vi "3kButtonsSys22x22.vi"() -> ()   [LabVIEW 2011]
doc: "3000 buttons from haobo.li@pansino.com.cn\nhttp://www.linkedin.com/pub/haobo-li/17/8a/220\nthanks to\nhttp://www.fatcow.com/free-icons"
panel:
  in  "Pansino 2":bool
  in  "Pansino":bool
  in  "zootool":bool
  in  "zoom_selection":bool
  in  "zoom_refresh":bool
  in  "zoom_out":bool
  in  "zoom_layer":bool
  in  "zoom_last":bool
  in  "zoom_in":bool
  in  "zoom_fit":bool
  in  "zoom_extend":bool
  in  "zoom_actual_equal":bool
  in  "zoom_actual":bool
  in  "zoom":bool
  in  "youtube":bool
  in  "yelp":bool
  in  "yellow_submarine":bool
  in  "yahoo_messenger":bool
  in  "yacht":bool
  in  "xing":bool
  in  "xhtml_valid":bool
  in  "xhtml_go":bool
  in  "xhtml_delete":bool
  in  "xhtml_add":bool
  in  "xhtml":bool
  in  "x_ray":bool
  in  "www_page":bool
  in  "wrench_orange":bool
  in  "wrench":bool
  in  "wrapping_tight":bool
  in  "wrapping_square":bool
  in  "wrapping_magazine":bool
  in  "wrapping_inline":bool
  in  "wrapping_in_front":bool
  in  "wrapping_edit":bool
  in  "wrapping_between":bool
  in  "wrapping_behind":bool
  in  "world_link":bool
  in  "world_go":bool
  in  "world_edit":bool
  in  "world_delete":bool
  in  "world_add":bool
  in  "world":bool
  in  "workspace":bool
  in  "wordpress_blog":bool
  in  "wordpress":bool
  in  "wizard_women":bool
  in  "wizard":bool
  in  "wishlist_add":bool
  in  "winrar_view":bool
  in  "winrar_extract":bool
  in  "winrar_add":bool
  in  "wine_pairings":bool
  in  "windy":bool
  in  "widgets":bool
  in  "widescreen":bool
  in  "whistle":bool
  in  "weight":bool
  in  "weighing_mashine":bool
  in  "webcam_error":bool
  in  "webcam_delete":bool
  in  "webcam_add":bool
  in  "webcam":bool
  in  "web_concierge":bool
  in  "weather_sun":bool
  in  "weather_snow":bool
  in  "weather_rain":bool
  in  "weather_lightning":bool
  in  "weather_cloudy":bool
  in  "weather_clouds":bool
  in  "wand":bool
  in  "wallet":bool
  in  "walk":bool
  in  "vslider":bool
  in  "vrule":bool
  in  "vlc":bool
  in  "visa_electron":bool
  in  "visa_2":bool
  in  "visa":bool
  in  "virus_protection":bool
  in  "virb":bool
  in  "vimeo":bool
  in  "viewstack":bool
  in  "videodisplay":bool
  in  "video_mode":bool
  in  "video":bool
  in  "viddler":bool
  in  "vhs":bool
  in  "vector_delete":bool
  in  "vector_add":bool
  in  "vector":bool
  in  "vdividedbox":bool
  in  "vcard_edit":bool
  in  "vcard_delete":bool
  in  "vcard_add":bool
  in  "vcard":bool
  in  "vbox":bool
  in  "user_zorro":bool
  in  "user_yoda":bool
  in  "user_wicket":bool
  in  "user_waiter_female_black":bool
  in  "user_waiter_female":bool
  in  "user_waiter":bool
  in  "user_viking_female":bool
  in  "user_viking":bool
  in  "user_vietnamese_female":bool
  in  "user_vietnamese":bool
  in  "user_trooper_captain":bool
  in  "user_trooper":bool
  in  "user_swimmer_female":bool
  in  "user_swimmer_black":bool
  in  "user_swimmer":bool
  in  "user_superman":bool
  in  "user_suit":bool
  in  "user_student_female_black":bool
  in  "user_student_female":bool
  in  "user_student_black":bool
  in  "user_student":bool
  in  "user_striper_black":bool
  in  "user_striper":bool
  in  "user_stewardess_black":bool
  in  "user_stewardess":bool
  in  "user_squidward":bool
  in  "user_sponge_bob":bool
  in  "user_spiderman":bool
  in  "user_soldier":bool
  in  "user_silhouette":bool
  in  "user_scream":bool
  in  "user_samurai":bool
  in  "user_sailor_black":bool
  in  "user_sailor":bool
  in  "user_robocop":bool
  in  "user_redskin":bool
  in  "user_red":bool
  in  "user_rambo":bool
  in  "user_racer":bool
  in  "user_r2d2":bool
  in  "user_queen_black":bool
  in  "user_queen":bool
  in  "user_pumpkin":bool
  in  "user_priest_black":bool
  in  "user_priest":bool
  in  "user_policeman_black":bool
  in  "user_policeman":bool
  in  "user_police_female_black":bool
  in  "user_police_female":bool
  in  "user_police_england":bool
  in  "user_plankton":bool
  in  "user_pirate":bool
  in  "user_pilot_civil":bool
  in  "user_pilot":bool
  in  "user_patrick":bool
  in  "user_orange":bool
  in  "user_oldwoman_black":bool
  in  "user_oldwoman":bool
  in  "user_oldman_black":bool
  in  "user_oldman":bool
  in  "user_officer_black":bool
  in  "user_officer":bool
  in  "user_nun_black":bool
  in  "user_nun":bool
  in  "user_nude_female_black":bool
  in  "user_nude_female":bool
  in  "user_nude_black":bool
  in  "user_nude":bool
  in  "user_ninja":bool
  in  "user_muslim_female":bool
  in  "user_muslim":bool
  in  "user_mexican":bool
  in  "user_medical_female_black":bool
  in  "user_medical_female":bool
  in  "user_medical_black":bool
  in  "user_medical":bool
  in  "user_maid":bool
  in  "user_lisa":bool
  in  "user_leprechaun":bool
  in  "user_knight":bool
  in  "user_king_black":bool
  in  "user_king":bool
  in  "user_judge_black":bool
  in  "user_judge":bool
  in  "user_jew":bool
  in  "user_jester":bool
  in  "user_jawa":bool
  in  "user_jason":bool
  in  "user_ironman":bool
  in  "user_indian_female":bool
  in  "user_indian":bool
  in  "user_imprisoned_female_black":bool
  in  "user_imprisoned_female":bool
  in  "user_imprisoned_black":bool
  in  "user_imprisoned":bool
  in  "user_hendrix":bool
  in  "user_halk":bool
  in  "user_green":bool
  in  "user_gray":bool
  in  "user_goth":bool
  in  "user_gomer":bool
  in  "user_go":bool
  in  "user_gladiator":bool
  in  "user_geisha":bool
  in  "user_freddy":bool
  in  "user_firefighter_black":bool
  in  "user_firefighter":bool
  in  "user_female":bool
  in  "user_eskimo_female":bool
  in  "user_eskimo":bool
  in  "user_emo":bool
  in  "user_egyptian_female":bool
  in  "user_egyptian":bool
  in  "user_edit":bool
  in  "user_dracula":bool
  in  "user_diver":bool
  in  "user_devil":bool
  in  "user_detective_gray":bool
  in  "user_detective":bool
  in  "user_delete":bool
  in  "user_death":bool
  in  "user_darth_vader":bool
  in  "user_crabs":bool
  in  "user_cowboy_female":bool
  in  "user_cowboy":bool
  in  "user_cook_female_black":bool
  in  "user_cook_female":bool
  in  "user_cook_black":bool
  in  "user_cook":bool
  in  "user_comment":bool
  in  "user_clown":bool
  in  "user_chief_female_black":bool
  in  "user_chief_female":bool
  in  "user_chief_black":bool
  in  "user_chief":bool
  in  "user_catwomen":bool
  in  "user_c3po":bool
  in  "user_buddhist":bool
  in  "user_boxer_black":bool
  in  "user_boxer":bool
  in  "user_blondy":bool
  in  "user_bishop":bool
  in  "user_bender":bool
  in  "user_beach_lifeguard_female":bool
  in  "user_beach_lifeguard":bool
  in  "user_batman":bool
  in  "user_bart":bool
  in  "user_banker":bool
  in  "user_ballplayer_black":bool
  in  "user_ballplayer":bool
  in  "user_astronaut":bool
  in  "user_angel_female_black":bool
  in  "user_angel_female":bool
  in  "user_angel_black":bool
  in  "user_angel":bool
  in  "user_alien":bool
  in  "user_add":bool
  in  "user":bool
  in  "usb_3":bool
  in  "update":bool
  in  "universal_binary":bool
  in  "unicorn":bool
  in  "understanding":bool
  in  "underle_dictionary":bool
  in  "umbrella":bool
  in  "ufo":bool
  in  "ubuntu":bool
  in  "twitter_2":bool
  in  "twitter_1":bool
  in  "tux":bool
  in  "turntable":bool
  in  "tumblr":bool
  in  "tubes":bool
  in  "tub":bool
  in  "trolley":bool
  in  "trojan_horse":bool
  in  "tree":bool
  in  "travel":bool
  in  "transmit_go":bool
  in  "transmit_error":bool
  in  "transmit_edit":bool
  in  "transmit_delete":bool
  in  "transmit_blue":bool
  in  "transmit_add":bool
  in  "transmit":bool
  in  "transform_shear":bool
  in  "transform_selection":bool
  in  "transform_scale":bool
  in  "transform_rotate_270":bool
  in  "transform_rotate_180":bool
  in  "transform_rotate_90":bool
  in  "transform_rotate":bool
  in  "transform_perspective":bool
  in  "transform_path":bool
  in  "transform_move":bool
  in  "transform_layer":bool
  in  "transform_flip":bool
  in  "transform_crop_resize":bool
  in  "transform_crop":bool
  in  "traffic_usage":bool
  in  "traffic_lights_yellow":bool
  in  "traffic_lights_red":bool
  in  "traffic_lights_green":bool
  in  "traffic_lights":bool
  in  "trade":bool
  in  "tractor":bool
  in  "toxic":bool
  in  "tower":bool
  in  "toucan":bool
  in  "total_plan_cost":bool
  in  "toster":bool
  in  "tornado":bool
  in  "torchere":bool
  in  "tooth":bool
  in  "toolbox":bool
  in  "to_do_list_cheked_all":bool
  in  "to_do_list_cheked_1":bool
  in  "to_do_list":bool
  in  "title_window":bool
  in  "tire":bool
  in  "tipper":bool
  in  "timeline_marker":bool
  in  "timeline":bool
  in  "time_go":bool
  in  "time_delete":bool
  in  "time_add":bool
  in  "time":bool
  in  "tilelist":bool
  in  "tick":bool
  in  "thumb_up":bool
  in  "thumb_down":bool
  in  "three_tags":bool
  in  "things_digital":bool
  in  "things_beauty":bool
  in  "theater":bool
  in  "textfield_rename":bool
  in  "textfield_key":bool
  in  "textfield_delete":bool
  in  "textfield_add":bool
  in  "textfield":bool
  in  "text_width":bool
  in  "text_uppercase":bool
  in  "text_underline":bool
  in  "text_superscript":bool
  in  "text_subscript":bool
  in  "text_strikethroungh":bool
  in  "text_smallcaps":bool
  in  "text_signature":bool
  in  "text_resize":bool
  in  "text_replace":bool
  in  "text_prose":bool
  in  "text_pagination_100":bool
  in  "text_pagination":bool
  in  "text_padding_top":bool
  in  "text_padding_right":bool
  in  "text_padding_left":bool
  in  "text_padding_bottom":bool
  in  "text_lowercase":bool
  in  "text_list_numbers":bool
  in  "text_list_bullets":bool
  in  "text_linespacing":bool
  in  "text_letterspacing":bool
  in  "text_letter_omega":bool
  in  "text_large_cap":bool
  in  "text_language":bool
  in  "text_kerning":bool
  in  "text_italic":bool
  in  "text_indent_remove":bool
  in  "text_indent":bool
  in  "text_horizontalrule":bool
  in  "text_heading_6":bool
  in  "text_heading_5":bool
  in  "text_heading_4":bool
  in  "text_heading_3":bool
  in  "text_heading_2":bool
  in  "text_heading_1":bool
  in  "text_dropcaps":bool
  in  "text_drama":bool
  in  "text_document_wrap":bool
  in  "text_document":bool
  in  "text_columns":bool
  in  "text_bold":bool
  in  "text_area":bool
  in  "text_allcaps":bool
  in  "text_align_right":bool
  in  "text_align_left":bool
  in  "text_align_justity":bool
  in  "text_align_center":bool
  in  "text":bool
  in  "terminal_seats_red":bool
  in  "terminal_seats_blue":bool
  in  "terminal":bool
  in  "temperature_5":bool
  in  "temperature_4":bool
  in  "temperature_3":bool
  in  "temperature_2":bool
  in  "temperature_1":bool
  in  "television_delete":bool
  in  "television_add":bool
  in  "television":bool
  in  "telephone_link":bool
  in  "telephone_key":bool
  in  "telephone_go":bool
  in  "telephone_error":bool
  in  "telephone_edit":bool
  in  "telephone_delete":bool
  in  "telephone_add":bool
  in  "telephone":bool
  in  "teddy_bear":bool
  in  "technorati":bool
  in  "teapot":bool
  in  "tea_cup":bool
  in  "tags_cloud":bool
  in  "tag_yellow":bool
  in  "tag_red":bool
  in  "tag_purple":bool
  in  "tag_pink":bool
  in  "tag_orange":bool
  in  "tag_green":bool
  in  "tag_blue_edit":bool
  in  "tag_blue_delete":bool
  in  "tag_blue_add":bool
  in  "tag_blue":bool
  in  "tag":bool
  in  "tabnavigator":bool
  in  "tablets":bool
  in  "table_torn":bool
  in  "table_tab_search":bool
  in  "table_tab_resize":bool
  in  "table_tab":bool
  in  "table_sum":bool
  in  "table_split":bool
  in  "table_sort":bool
  in  "table_sheet":bool
  in  "table_select_row":bool
  in  "table_select_column":bool
  in  "table_select_big":bool
  in  "table_select_all":bool
  in  "table_select":bool
  in  "table_save":bool
  in  "table_row_insert":bool
  in  "table_row_delete":bool
  in  "table_replace":bool
  in  "table_relationship":bool
  in  "table_refresh":bool
  in  "table_paint_can":bool
  in  "table_multiple":bool
  in  "table_money":bool
  in  "table_link":bool
  in  "table_lightning":bool
  in  "table_key":bool
  in  "table_insert":bool
  in  "table_import":bool
  in  "table_heatmap":bool
  in  "table_go":bool
  in  "table_gear":bool
  in  "table_export":bool
  in  "table_excel":bool
  in  "table_error":bool
  in  "table_edit":bool
  in  "table_delete":bool
  in  "table_chart":bool
  in  "table_add":bool
  in  "table":bool
  in  "tabbar":bool
  in  "tab_go":bool
  in  "tab_edit":bool
  in  "tab_delete":bool
  in  "tab_add":bool
  in  "tab":bool
  in  "system_time":bool
  in  "system_monitor":bool
  in  "sword":bool
  in  "switch_220v":bool
  in  "switch_120v":bool
  in  "switch":bool
  in  "swf_loader":bool
  in  "support":bool
  in  "sun_rain":bool
  in  "sun_cloudy":bool
  in  "sum":bool
  in  "subwoofer":bool
  in  "style_go":bool
  in  "style_edit":bool
  in  "style_delete":bool
  in  "style_add":bool
  in  "style":bool
  in  "stumble_upon":bool
  in  "street_stall":bool
  in  "storage":bool
  in  "stopwatch_start":bool
  in  "stopwatch_pause":bool
  in  "stopwatch_finish":bool
  in  "stop":bool
  in  "stethoscope_vintage":bool
  in  "stethoscope":bool
  in  "steering_wheel_3":bool
  in  "steering_wheel_2":bool
  in  "steering_wheel":bool
  in  "steak_meat":bool
  in  "steak_fish":bool
  in  "status_online":bool
  in  "status_offline":bool
  in  "status_busy":bool
  in  "status_away":bool
  in  "statistics":bool
  in  "star":bool
  in  "stamp_pattern":bool
  in  "ssl_certificates":bool
  in  "sql_join_right_exclude":bool
  in  "sql_join_right":bool
  in  "sql_join_outer_exclude":bool
  in  "sql_join_outer":bool
  in  "sql_join_left_exclude":bool
  in  "sql_join_left":bool
  in  "sql_join_inner":bool
  in  "sql_join":bool
  in  "spring":bool
  in  "sport_tennis":bool
  in  "sport_soccer":bool
  in  "sport_shuttlecock":bool
  in  "sport_raquet":bool
  in  "sport_golf":bool
  in  "sport_football":bool
  in  "sport_basketball":bool
  in  "sport_8ball":bool
  in  "sport":bool
  in  "spill":bool
  in  "spider_web":bool
  in  "spellcheck_error":bool
  in  "spellcheck":bool
  in  "speedometer":bool
  in  "speakers":bool
  in  "spam_filter":bool
  in  "spam":bool
  in  "spacer":bool
  in  "source_code":bool
  in  "soup":bool
  in  "sound_none":bool
  in  "sound_mute":bool
  in  "sound_low":bool
  in  "sound_delete":bool
  in  "sound_add":bool
  in  "sound":bool
  in  "sort_descending":bool
  in  "sort_columns":bool
  in  "sort_ascending":bool
  in  "solar":bool
  in  "soil_layers":bool
  in  "soap":bool
  in  "snowman":bool
  in  "snow_rain":bool
  in  "sneakers":bool
  in  "snapshot":bool
  in  "snake_and_cup":bool
  in  "snail":bool
  in  "small_tiles":bool
  in  "small_car":bool
  in  "small_business":bool
  in  "slideshow":bool
  in  "slackware":bool
  in  "skype":bool
  in  "skins":bool
  in  "skate":bool
  in  "size_vertical":bool
  in  "size_horizontal":bool
  in  "sitemap_color":bool
  in  "sitemap":bool
  in  "site_enhancer":bool
  in  "site_backup_and_restore":bool
  in  "siren":bool
  in  "sign":bool
  in  "shuriken":bool
  in  "showel":bool
  in  "shorts":bool
  in  "shopping":bool
  in  "shop_open":bool
  in  "shop_closed":bool
  in  "shirt_polo":bool
  in  "shield_go":bool
  in  "shield_delete":bool
  in  "shield_add":bool
  in  "shield":bool
  in  "sheduled_task":bool
  in  "sharpen":bool
  in  "share":bool
  in  "shape_ungroup":bool
  in  "shape_square_link":bool
  in  "shape_square_key":bool
  in  "shape_square_go":bool
  in  "shape_square_error":bool
  in  "shape_square_edit":bool
  in  "shape_square_delete":bool
  in  "shape_square_add":bool
  in  "shape_square":bool
  in  "shape_rotate_clockwise":bool
  in  "shape_rotate_anticlockwise":bool
  in  "shape_move_front":bool
  in  "shape_move_forwards":bool
  in  "shape_move_backwards":bool
  in  "shape_move_back":bool
  in  "shape_handles":bool
  in  "shape_group":bool
  in  "shape_flip_vertical":bool
  in  "shape_flip_horizontal":bool
  in  "shape_align_top":bool
  in  "shape_align_right":bool
  in  "shape_align_middle":bool
  in  "shape_align_left":bool
  in  "shape_align_center":bool
  in  "shape_align_bottom":bool
  in  "shading":bool
  in  "setting_tools":bool
  in  "set_security_question":bool
  in  "session_idle_time":bool
  in  "server_uncompress":bool
  in  "server_stanchion":bool
  in  "server_link":bool
  in  "server_lightning":bool
  in  "server_key":bool
  in  "server_information":bool
  in  "server_go":bool
  in  "server_error":bool
  in  "server_edit":bool
  in  "server_delete":bool
  in  "server_database":bool
  in  "server_connect":bool
  in  "server_compress":bool
  in  "server_components":bool
  in  "server_chart":bool
  in  "server_add":bool
  in  "server":bool
  in  "sertificate":bool
  in  "select_restangular":bool
  in  "select_lasso":bool
  in  "select_invert":bool
  in  "select_ellipse":bool
  in  "select_continuous_area":bool
  in  "select_by_intersection":bool
  in  "select_by_difference":bool
  in  "select_by_color":bool
  in  "select_by_adding_to_selection":bool
  in  "select":bool
  in  "search_plus":bool
  in  "search_minus":bool
  in  "scull":bool
  in  "scroller_bar":bool
  in  "scripts":bool
  in  "script_yellow":bool
  in  "script_torn":bool
  in  "script_save":bool
  in  "script_red":bool
  in  "script_palette":bool
  in  "script_link":bool
  in  "script_lightning":bool
  in  "script_key":bool
  in  "script_green":bool
  in  "script_go":bool
  in  "script_gear":bool
  in  "script_error":bool
  in  "script_edit":bool
  in  "script_delete":bool
  in  "script_code_red":bool
  in  "script_code":bool
  in  "script_black":bool
  in  "script_add":bool
  in  "script":bool
  in  "screwdriver":bool
  in  "screen_error":bool
  in  "scanner":bool
  in  "scalpel":bool
  in  "scale_image":bool
  in  "save_money":bool
  in  "save_as":bool
  in  "satellite_dish":bool
  in  "satellite":bool
  in  "santa":bool
  in  "salver":bool
  in  "sallary_deferrais":bool
  in  "safe":bool
  in  "safari_browser":bool
  in  "ruby_put":bool
  in  "ruby_link":bool
  in  "ruby_key":bool
  in  "ruby_go":bool
  in  "ruby_get":bool
  in  "ruby_gear":bool
  in  "ruby_delete":bool
  in  "ruby_add":bool
  in  "ruby":bool
  in  "rubber_duck":bool
  in  "rss_valid":bool
  in  "rss_go":bool
  in  "rss_delete":bool
  in  "rss_add":bool
  in  "rss":bool
  in  "routing_turning_right":bool
  in  "routing_turning_left":bool
  in  "routing_turnaround_right":bool
  in  "routing_turnaround_left":bool
  in  "routing_turn_u":bool
  in  "routing_turn_right_2":bool
  in  "routing_turn_right":bool
  in  "routing_turn_left_crossroads":bool
  in  "routing_turn_left_2":bool
  in  "routing_turn_left":bool
  in  "routing_turn_arround_right":bool
  in  "routing_turn_arround_left":bool
  in  "routing_intersection_right":bool
  in  "routing_go_straight_right":bool
  in  "routing_go_straight_left":bool
  in  "routing_go_right":bool
  in  "routing_go_left":bool
  in  "routing_forward":bool
  in  "routing_around":bool
  in  "router":bool
  in  "rotate_90":bool
  in  "rosette":bool
  in  "role":bool
  in  "rocking_chair":bool
  in  "robo_to":bool
  in  "roadworks":bool
  in  "road_sign":bool
  in  "rip":bool
  in  "ring":bool
  in  "richtext_editor":bool
  in  "ribbon":bool
  in  "resultset_previous":bool
  in  "resultset_next":bool
  in  "resultset_last":bool
  in  "resultset_first":bool
  in  "restaurant_menu":bool
  in  "resources":bool
  in  "resource_usage":bool
  in  "resize_picture":bool
  in  "reseller_programm":bool
  in  "reseller_account_template":bool
  in  "reseller_account":bool
  in  "report_word":bool
  in  "report_user":bool
  in  "report_torn":bool
  in  "report_picture":bool
  in  "report_magnify":bool
  in  "report_link":bool
  in  "report_key":bool
  in  "report_go":bool
  in  "report_edit":bool
  in  "report_disk":bool
  in  "report_delete":bool
  in  "report_add":bool
  in  "report":bool
  in  "remote":bool
  in  "reddit":bool
  in  "red_line":bool
  in  "recycle_bag":bool
  in  "recycle":bool
  in  "real_estate":bool
  in  "readernaut":bool
  in  "rainbow_cloud":bool
  in  "rainbow":bool
  in  "rain":bool
  in  "radiolocator":bool
  in  "radiobutton_group":bool
  in  "radiobutton":bool
  in  "radioactivity":bool
  in  "radio_2":bool
  in  "radio_1":bool
  in  "rabbit":bool
  in  "question":bool
  in  "qip_online":bool
  in  "qip_offline":bool
  in  "qip_occupied":bool
  in  "qip_not_available":bool
  in  "qip_invisible_for_all":bool
  in  "qip_invisible":bool
  in  "qip_free_for_chat":bool
  in  "qip_eating":bool
  in  "qip_dnd":bool
  in  "qip_bad_mood":bool
  in  "qip_away":bool
  in  "qip_at_work":bool
  in  "qip_at_home":bool
  in  "qip_angry":bool
  in  "qik":bool
  in  "purse":bool
  in  "progressbar":bool
  in  "profiles":bool
  in  "production_copyleft":bool
  in  "processor":bool
  in  "private":bool
  in  "printer_error":bool
  in  "printer_empty":bool
  in  "printer_delete":bool
  in  "printer_add":bool
  in  "printer":bool
  in  "print_size":bool
  in  "price_watch":bool
  in  "price_comparison":bool
  in  "price_alert":bool
  in  "premium_support":bool
  in  "preferences":bool
  in  "power_surge":bool
  in  "posterous":bool
  in  "postage_stamp":bool
  in  "port":bool
  in  "popcorn":bool
  in  "pop_mail":bool
  in  "poo":bool
  in  "poker":bool
  in  "plurk":bool
  in  "plugin_link":bool
  in  "plugin_go":bool
  in  "plugin_error":bool
  in  "plugin_edit":bool
  in  "plugin_disabled":bool
  in  "plugin_delete":bool
  in  "plugin_add":bool
  in  "plugin":bool
  in  "plotchart":bool
  in  "playstation":bool
  in  "Plant":bool
  in  "plane":bool
  in  "places":bool
  in  "pizza":bool
  in  "pirate_flag":bool
  in  "pint":bool
  in  "pill_go":bool
  in  "pill_delete":bool
  in  "pill_add":bool
  in  "pill":bool
  in  "pilcrow":bool
  in  "piechart":bool
  in  "piece_of_cake":bool
  in  "pictures":bool
  in  "picture_save":bool
  in  "picture_link":bool
  in  "picture_key":bool
  in  "picture_go":bool
  in  "picture_frame":bool
  in  "picture_error":bool
  in  "picture_empty":bool
  in  "picture_edit":bool
  in  "picture_delete":bool
  in  "picture_add":bool
  in  "picture":bool
  in  "picasa":bool
  in  "piano":bool
  in  "pi_math":bool
  in  "photos":bool
  in  "photo_link":bool
  in  "photo_delete":bool
  in  "photo_add":bool
  in  "photo":bool
  in  "phone_vintage":bool
  in  "phone_sound":bool
  in  "phone_delete":bool
  in  "phone_Android":bool
  in  "phone_add":bool
  in  "phone":bool
  in  "personals":bool
  in  "personal_finance":bool
  in  "perfomance":bool
  in  "pepper":bool
  in  "pencil_go":bool
  in  "pencil_delete":bool
  in  "pencil_add":bool
  in  "pencil":bool
  in  "pearl":bool
  in  "peak_cap":bool
  in  "peacock":bool
  in  "pci":bool
  in  "pc_linux_os":bool
  in  "paypal-2":bool
  in  "paypal":bool
  in  "paste_word":bool
  in  "paste_plain":bool
  in  "participation_rate":bool
  in  "parrot":bool
  in  "paper_airplane":bool
  in  "panel":bool
  in  "pandora":bool
  in  "palette":bool
  in  "paintcan":bool
  in  "paintbrush":bool
  in  "page_world":bool
  in  "page_word":bool
  in  "page_white_zip":bool
  in  "page_white_wrench":bool
  in  "page_white_world":bool
  in  "page_white_word":bool
  in  "page_white_width":bool
  in  "page_white_visualstudio":bool
  in  "page_white_vector":bool
  in  "page_white_tux":bool
  in  "page_white_text_width":bool
  in  "page_white_text":bool
  in  "page_white_star":bool
  in  "page_white_stack":bool
  in  "page_white_ruby":bool
  in  "page_white_put":bool
  in  "page_white_powerpoint":bool
  in  "page_white_picture":bool
  in  "page_white_php":bool
  in  "page_white_paste":bool
  in  "page_white_paintbrush":bool
  in  "page_white_paint":bool
  in  "page_white_office":bool
  in  "page_white_medal":bool
  in  "page_white_magnify":bool
  in  "page_white_link":bool
  in  "page_white_lightning":bool
  in  "page_white_key":bool
  in  "page_white_horizontal":bool
  in  "page_white_h":bool
  in  "page_white_go":bool
  in  "page_white_get":bool
  in  "page_white_gear":bool
  in  "page_white_flash":bool
  in  "page_white_find":bool
  in  "page_white_excel":bool
  in  "page_white_error":bool
  in  "page_white_edit":bool
  in  "page_white_dvd":bool
  in  "page_white_delete":bool
  in  "page_white_database":bool
  in  "page_white_cup":bool
  in  "page_white_csharp":bool
  in  "page_white_cplusplus":bool
  in  "page_white_copy":bool
  in  "page_white_compress":bool
  in  "page_white_code_red":bool
  in  "page_white_code":bool
  in  "page_white_cd":bool
  in  "page_white_camera":bool
  in  "page_white_c":bool
  in  "page_white_add":bool
  in  "page_white_actionscript":bool
  in  "page_white_acrobat":bool
  in  "page_white":bool
  in  "page_save":bool
  in  "page_refresh":bool
  in  "page_red":bool
  in  "page_paste":bool
  in  "page_paintbrush":bool
  in  "page_magnifier":bool
  in  "page_link":bool
  in  "page_lightning":bool
  in  "page_key":bool
  in  "page_green":bool
  in  "page_go":bool
  in  "page_gear":bool
  in  "page_find":bool
  in  "page_excel":bool
  in  "page_error":bool
  in  "page_edit":bool
  in  "page_delete":bool
  in  "page_copy":bool
  in  "page_code":bool
  in  "page_attach":bool
  in  "page_add":bool
  in  "page":bool
  in  "package_link":bool
  in  "package_green":bool
  in  "package_go":bool
  in  "package_delete":bool
  in  "package_add":bool
  in  "package":bool
  in  "other_phone":bool
  in  "orthodox_church":bool
  in  "ornament_gold":bool
  in  "orkut":bool
  in  "origami":bool
  in  "orbit":bool
  in  "opera":bool
  in  "openid":bool
  in  "open_suse":bool
  in  "open_folder":bool
  in  "omelet":bool
  in  "oil":bool
  in  "numeric_stepper":bool
  in  "note_torn":bool
  in  "note_go":bool
  in  "note_error":bool
  in  "note_edit":bool
  in  "note_delete":bool
  in  "note_add":bool
  in  "note":bool
  in  "non_derivative":bool
  in  "nokia_s60":bool
  in  "node-tree":bool
  in  "no_smoking":bool
  in  "no_requirements":bool
  in  "no_image":bool
  in  "no_drm_trm":bool
  in  "no_commercial":bool
  in  "newsvine":bool
  in  "newspaper_link":bool
  in  "newspaper_go":bool
  in  "newspaper_delete":bool
  in  "newspaper_add":bool
  in  "newspaper":bool
  in  "new":bool
  in  "network-share":bool
  in  "networking_red":bool
  in  "networking_green":bool
  in  "networking":bool
  in  "network_wireless":bool
  in  "network_ip":bool
  in  "network_hub":bool
  in  "network_folder":bool
  in  "network_firewall":bool
  in  "network_ethernet":bool
  in  "network_clouds":bool
  in  "network_cloud":bool
  in  "network_adapter":bool
  in  "netvibes":bool
  in  "nameboard_open":bool
  in  "myspace":bool
  in  "my_name_is_e":bool
  in  "mustache":bool
  in  "music":bool
  in  "multitool":bool
  in  "multiplied_by_100":bool
  in  "multiplied_by_10":bool
  in  "multiplied_by_5":bool
  in  "multiplied_by_3":bool
  in  "multiplied_by_2":bool
  in  "msn_messenger":bool
  in  "ms_frontpage":bool
  in  "ms_exchange":bool
  in  "movies":bool
  in  "move_to_folder":bool
  in  "mouse_select_scroll":bool
  in  "mouse_select_right":bool
  in  "mouse_select_left":bool
  in  "mouse_error":bool
  in  "mouse_delete":bool
  in  "mouse_add":bool
  in  "mouse_2":bool
  in  "mouse":bool
  in  "motherboard":bool
  in  "mosque":bool
  in  "moon":bool
  in  "monitor_window_3d":bool
  in  "monitor_window":bool
  in  "monitor_wallpaper":bool
  in  "monitor_sidebar":bool
  in  "monitor_screensaver":bool
  in  "monitor_link":bool
  in  "monitor_lightning":bool
  in  "monitor_go":bool
  in  "monitor_error":bool
  in  "monitor_edit":bool
  in  "monitor_delete":bool
  in  "monitor_add":bool
  in  "monitor":bool
  in  "moneybox":bool
  in  "money_yen":bool
  in  "money_pound":bool
  in  "money_in_envelope":bool
  in  "money_euro":bool
  in  "money_dollar":bool
  in  "money_delete":bool
  in  "money_bookers":bool
  in  "money_bag":bool
  in  "money_add":bool
  in  "money":bool
  in  "molecule":bool
  in  "mobile_me":bool
  in  "mixx":bool
  in  "mixture":bool
  in  "mixer":bool
  in  "milestone":bool
  in  "microwave":bool
  in  "microscope":bool
  in  "microphone":bool
  in  "microformats":bool
  in  "micro_sd_blue":bool
  in  "micro_sd":bool
  in  "metronome":bool
  in  "metro":bool
  in  "messenger":bool
  in  "menubar":bool
  in  "menu_item":bool
  in  "menu":bool
  in  "medical_record":bool
  in  "medal_silver_delete":bool
  in  "medal_silver_add":bool
  in  "medal_silver_3":bool
  in  "medal_silver_2":bool
  in  "medal_silver_1":bool
  in  "medal_gold_delete":bool
  in  "medal_gold_add":bool
  in  "medal_gold_3":bool
  in  "medal_gold_2":bool
  in  "medal_gold_1":bool
  in  "medal_bronze_delete":bool
  in  "medal_bronze_add":bool
  in  "medal_bronze_3":bool
  in  "medal_bronze_2":bool
  in  "medal_bronze_1":bool
  in  "medal_award_silver":bool
  in  "medal_award_gold":bool
  in  "medal_award_bronze":bool
  in  "measure_crop":bool
  in  "measure":bool
  in  "master_card":bool
  in  "mask":bool
  in  "marketwatch":bool
  in  "mario":bool
  in  "map_torn":bool
  in  "map_magnify":bool
  in  "map_go":bool
  in  "map_edit":bool
  in  "map_delete":bool
  in  "map_add":bool
  in  "map":bool
  in  "mandriva":bool
  in  "male":bool
  in  "mail-trash":bool
  in  "mail_yellow":bool
  in  "mail_torn":bool
  in  "mail_server_setting":bool
  in  "mail_red":bool
  in  "mail_green":bool
  in  "mail_box":bool
  in  "mail_black":bool
  in  "magnifier_zoom_out":bool
  in  "magnifier_zoom_in":bool
  in  "magnifier":bool
  in  "magnet":bool
  in  "magic_wand_2":bool
  in  "luggage_brown_tag":bool
  in  "luggage_brown":bool
  in  "luggage":bool
  in  "lorry_link":bool
  in  "lorry_go":bool
  in  "lorry_flatbed":bool
  in  "lorry_error":bool
  in  "lorry_delete":bool
  in  "lorry_add":bool
  in  "lorry":bool
  in  "lollypop":bool
  in  "lollipop":bool
  in  "lock_open":bool
  in  "lock_go":bool
  in  "lock_edit":bool
  in  "lock_delete":bool
  in  "lock_break":bool
  in  "lock_add":bool
  in  "lock":bool
  in  "location_pin":bool
  in  "locate":bool
  in  "livejournal":bool
  in  "list":bool
  in  "linux_mint":bool
  in  "linkedin":bool
  in  "linkbar":bool
  in  "link_unchain":bool
  in  "link_juice":bool
  in  "link_go":bool
  in  "link_edit":bool
  in  "link_delete":bool
  in  "link_button":bool
  in  "link_break":bool
  in  "link_add":bool
  in  "link":bool
  in  "linechart":bool
  in  "line_split":bool
  in  "lightning_go":bool
  in  "lightning_delete":bool
  in  "lightning_add":bool
  in  "lightning":bool
  in  "lighthouse_shine":bool
  in  "lighthouse":bool
  in  "lightbulb_off":bool
  in  "lightbulb_delete":bool
  in  "lightbulb_add":bool
  in  "lightbulb":bool
  in  "light_circle_green":bool
  in  "life_vest":bool
  in  "license_management":bool
  in  "license_key":bool
  in  "legend":bool
  in  "led":bool
  in  "layouts_split_vertical":bool
  in  "layouts_split":bool
  in  "layouts_select_sidebar":bool
  in  "layouts_select_footer":bool
  in  "layouts_select_content":bool
  in  "layouts_select":bool
  in  "layouts_join_vertical":bool
  in  "layouts_join":bool
  in  "layouts_hf_3":bool
  in  "layouts_hf_2_equal":bool
  in  "layouts_header_footer_3":bool
  in  "layouts_header_footer_2":bool
  in  "layouts_header_footer":bool
  in  "layouts_header_3_mix":bool
  in  "layouts_header_3":bool
  in  "layouts_header_2_equal":bool
  in  "layouts_header_2":bool
  in  "layouts_header":bool
  in  "layouts_design":bool
  in  "layouts_6":bool
  in  "layouts_4":bool
  in  "layouts_3_mix":bool
  in  "layouts_3":bool
  in  "layouts_2":bool
  in  "layouts":bool
  in  "layout_sidebar":bool
  in  "layout_link":bool
  in  "layout_header":bool
  in  "layout_error":bool
  in  "layout_edit":bool
  in  "layout_delete":bool
  in  "layout_content":bool
  in  "layout_add":bool
  in  "layout":bool
  in  "layers_map":bool
  in  "layers":bool
  in  "layer_wms":bool
  in  "layer_vector":bool
  in  "layer_transparent":bool
  in  "layer_to_image_size":bool
  in  "layer_stack_arrange_back":bool
  in  "layer_stack_arrange":bool
  in  "layer_shred":bool
  in  "layer_shape_text":bool
  in  "layer_shape_round":bool
  in  "layer_shape_polyline":bool
  in  "layer_shape_ellipse":bool
  in  "layer_shape":bool
  in  "layer_shaded_relief":bool
  in  "layer_shade":bool
  in  "layer_select":bool
  in  "layer_save":bool
  in  "layer_rgb":bool
  in  "layer_resize_replicate_v":bool
  in  "layer_resize_replicate_h":bool
  in  "layer_resize_actual":bool
  in  "layer_resize":bool
  in  "layer_remove":bool
  in  "layer_redraw":bool
  in  "layer_raster_3d":bool
  in  "layer_raster":bool
  in  "layer_open":bool
  in  "layer_mask":bool
  in  "layer_label":bool
  in  "layer_import":bool
  in  "layer_histogram":bool
  in  "layer_his":bool
  in  "layer_group":bool
  in  "layer_grid":bool
  in  "layer_gps":bool
  in  "layer_export":bool
  in  "layer_edit":bool
  in  "layer_delete":bool
  in  "layer_database":bool
  in  "layer_create":bool
  in  "layer_command":bool
  in  "layer_chart":bool
  in  "layer_cell_cats":bool
  in  "layer_aspect_arrow":bool
  in  "layer_arrange_back":bool
  in  "layer_arrange":bool
  in  "layer_add":bool
  in  "layer":bool
  in  "last_fm":bool
  in  "large_tiles":bool
  in  "laptop":bool
  in  "language":bool
  in  "landmarks":bool
  in  "ladybird":bool
  in  "knot":bool
  in  "kids":bool
  in  "keyboard_magnify":bool
  in  "keyboard_delete":bool
  in  "keyboard_add":bool
  in  "keyboard":bool
  in  "key_z":bool
  in  "key_y":bool
  in  "key_x":bool
  in  "key_w":bool
  in  "key_v":bool
  in  "key_u":bool
  in  "key_t":bool
  in  "key_solid":bool
  in  "key_s":bool
  in  "key_r":bool
  in  "key_q":bool
  in  "key_p":bool
  in  "key_o":bool
  in  "key_n":bool
  in  "key_m":bool
  in  "key_l":bool
  in  "key_k":bool
  in  "key_j":bool
  in  "key_i":bool
  in  "key_h":bool
  in  "key_go":bool
  in  "key_g":bool
  in  "key_f":bool
  in  "key_escape":bool
  in  "key_e":bool
  in  "key_delete":bool
  in  "key_d":bool
  in  "key_c":bool
  in  "key_b":bool
  in  "key_add":bool
  in  "key_a":bool
  in  "key":bool
  in  "json":bool
  in  "joystick_error":bool
  in  "joystick_delete":bool
  in  "joystick_add":bool
  in  "joystick":bool
  in  "jeans":bool
  in  "jason_mask":bool
  in  "jar_open":bool
  in  "jar_empty":bool
  in  "jacket":bool
  in  "italy":bool
  in  "ipod_sound":bool
  in  "ipod_cast_delete":bool
  in  "ipod_cast_add":bool
  in  "ipod_cast":bool
  in  "ipod":bool
  in  "iphone":bool
  in  "ipad":bool
  in  "ip_class":bool
  in  "ip_block":bool
  in  "ip":bool
  in  "investment_menu_quality":bool
  in  "internet_explorer":bool
  in  "interface_preferences":bool
  in  "installer_box":bool
  in  "insert_object":bool
  in  "insert_element":bool
  in  "injection":bool
  in  "information":bool
  in  "info_rhombus":bool
  in  "index-cards":bool
  in  "inbox_upload":bool
  in  "inbox_table":bool
  in  "inbox_slide":bool
  in  "inbox_images":bool
  in  "inbox_film":bool
  in  "inbox_empty":bool
  in  "inbox_download":bool
  in  "inbox_document_text":bool
  in  "inbox_document_music":bool
  in  "inbox_document":bool
  in  "images_flickr":bool
  in  "images":bool
  in  "image_link":bool
  in  "image_edit":bool
  in  "image_delete":bool
  in  "image_add":bool
  in  "image":bool
  in  "im_messenger":bool
  in  "ilike":bool
  in  "icecream":bool
  in  "ice_cube":bool
  in  "hummingbird":bool
  in  "http_status_unavailable":bool
  in  "http_status_temporary":bool
  in  "http_status_server_error":bool
  in  "http_status_permanent":bool
  in  "http_status_ok_success":bool
  in  "http_status_not_found":bool
  in  "html_valid":bool
  in  "html_go":bool
  in  "html_delete":bool
  in  "html_add":bool
  in  "html_5":bool
  in  "html":bool
  in  "hslider":bool
  in  "hrule":bool
  in  "house_two":bool
  in  "house_one":bool
  in  "house_link":bool
  in  "house_go":bool
  in  "house":bool
  in  "hourglass_link":bool
  in  "hourglass_go":bool
  in  "hourglass_delete":bool
  in  "hourglass_add":bool
  in  "hourglass":bool
  in  "hotjobs":bool
  in  "hot":bool
  in  "hostname":bool
  in  "hospital":bool
  in  "horoscopes":bool
  in  "horn":bool
  in  "horizontal_list":bool
  in  "home_page":bool
  in  "holly":bool
  in  "hlocchart":bool
  in  "hippocampus":bool
  in  "highlighter_text":bool
  in  "highlighter":bool
  in  "help":bool
  in  "helmet_mine":bool
  in  "helmet":bool
  in  "helicopter":bool
  in  "heart_half":bool
  in  "heart_empty":bool
  in  "heart_delete":bool
  in  "heart_break":bool
  in  "heart_add":bool
  in  "heart":bool
  in  "health":bool
  in  "headphone_mic":bool
  in  "headphone":bool
  in  "hdividedbox":bool
  in  "hd_ready":bool
  in  "hd_1080":bool
  in  "hd_720":bool
  in  "hbox":bool
  in  "hat":bool
  in  "hardware_building_oem":bool
  in  "handbag":bool
  in  "hand_property":bool
  in  "hand_point_270":bool
  in  "hand_point_180":bool
  in  "hand_point_090":bool
  in  "hand_point":bool
  in  "hand_ily":bool
  in  "hand_fuck":bool
  in  "hand":bool
  in  "hammer":bool
  in  "hamburger":bool
  in  "half_moon":bool
  in  "gun":bool
  in  "group_link":bool
  in  "group_key":bool
  in  "group_go":bool
  in  "group_gear":bool
  in  "group_error":bool
  in  "group_edit":bool
  in  "group_delete":bool
  in  "group_add":bool
  in  "group":bool
  in  "grooveshark":bool
  in  "grid":bool
  in  "grenade":bool
  in  "green_yellow":bool
  in  "green_wormhole":bool
  in  "green":bool
  in  "grass":bool
  in  "gps_handheld":bool
  in  "gps_automotive":bool
  in  "gowalla":bool
  in  "google_webmaster_tools":bool
  in  "google_web_elements":bool
  in  "google_wave":bool
  in  "google_voice":bool
  in  "google_talk":bool
  in  "google_plus":bool
  in  "google_new":bool
  in  "google_map_satellite":bool
  in  "google_map":bool
  in  "google_custom_search":bool
  in  "google_adsense":bool
  in  "google":bool
  in  "globe_place":bool
  in  "globe_network":bool
  in  "globe_model":bool
  in  "global_telecom":bool
  in  "glass_narrow":bool
  in  "gift_add":bool
  in  "geotag":bool
  in  "georectify":bool
  in  "gentoo_linux":bool
  in  "gear_in":bool
  in  "gcp_rms":bool
  in  "gcp":bool
  in  "gas":bool
  in  "gamespot":bool
  in  "game_monitor":bool
  in  "ftp":bool
  in  "fruit_lime":bool
  in  "fruit_grape":bool
  in  "friendfeed":bool
  in  "freebsd":bool
  in  "forrst":bool
  in  "formheading":bool
  in  "form":bool
  in  "forklift":bool
  in  "font_superscript":bool
  in  "font_subscript":bool
  in  "font_red_delete":bool
  in  "font_red":bool
  in  "font_go":bool
  in  "font_delete":bool
  in  "font_colors":bool
  in  "font_add":bool
  in  "font":bool
  in  "folding_fan":bool
  in  "folders_explorer":bool
  in  "folders":bool
  in  "folder_wrench":bool
  in  "folder_vertical_zipper":bool
  in  "folder_vertical_torn":bool
  in  "folder_vertical_rename":bool
  in  "folder_vertical_open":bool
  in  "folder_vertical_document":bool
  in  "folder_user":bool
  in  "folder_torn":bool
  in  "folder_table":bool
  in  "folder_star":bool
  in  "folder_stand":bool
  in  "folder_search":bool
  in  "folder_red":bool
  in  "folder_picture":bool
  in  "folder_palette":bool
  in  "folder_page_white":bool
  in  "folder_page":bool
  in  "folder_link":bool
  in  "folder_lightbulb":bool
  in  "folder_key":bool
  in  "folder_image":bool
  in  "folder_heart":bool
  in  "folder_green":bool
  in  "folder_go":bool
  in  "folder_find":bool
  in  "folder_feed":bool
  in  "folder_explore":bool
  in  "folder_error":bool
  in  "folder_edit":bool
  in  "folder_delete":bool
  in  "folder_database":bool
  in  "folder_camera":bool
  in  "folder_bug":bool
  in  "folder_brick":bool
  in  "folder_blue":bool
  in  "folder_black":bool
  in  "folder_bell":bool
  in  "folder_add":bool
  in  "folder":bool
  in  "fog":bool
  in  "flower":bool
  in  "flood_it":bool
  in  "flickr":bool
  in  "flex_builder":bool
  in  "flex":bool
  in  "flask_empty":bool
  in  "flask":bool
  in  "flashlight_shine":bool
  in  "flashlight":bool
  in  "flashdisk":bool
  in  "flamingo":bool
  in  "flag_zimbabwe":bool
  in  "flag_zambia":bool
  in  "flag_yemen":bool
  in  "flag_yellow":bool
  in  "flag_wwf":bool
  in  "flag_wto":bool
  in  "flag_wallis_and_futuna":bool
  in  "flag_wales":bool
  in  "flag_virgin_islands":bool
  in  "flag_vietnam":bool
  in  "flag_venezuela":bool
  in  "flag_vatican_city":bool
  in  "flag_vanuatu":bool
  in  "flag_uzbekistan":bool
  in  "flag_usa":bool
  in  "flag_uruquay":bool
  in  "flag_united_nations":bool
  in  "flag_united_arab_emirates":bool
  in  "flag_unesco":bool
  in  "flag_ukraine":bool
  in  "flag_uganda":bool
  in  "flag_tuvalu":bool
  in  "flag_turks_and_caicos_islands":bool
  in  "flag_turkmenistan":bool
  in  "flag_turkey":bool
  in  "flag_tunisia":bool
  in  "flag_trinidad_and_tobago":bool
  in  "flag_tonga":bool
  in  "flag_togo":bool
  in  "flag_tibet":bool
  in  "flag_thailand":bool
  in  "flag_tanzania":bool
  in  "flag_tajikistan":bool
  in  "flag_taiwan":bool
  in  "flag_syria":bool
  in  "flag_switzerland":bool
  in  "flag_sweden":bool
  in  "flag_swaziland":bool
  in  "flag_suriname":bool
  in  "flag_sudan":bool
  in  "flag_sri_lanka":bool
  in  "flag_spain":bool
  in  "flag_south_korea":bool
  in  "flag_south_georgia":bool
  in  "flag_south_africa":bool
  in  "flag_somalia":bool
  in  "flag_solomon_islands":bool
  in  "flag_slovenia":bool
  in  "flag_slovakia":bool
  in  "flag_singapore":bool
  in  "flag_sierra_leone":bool
  in  "flag_seychelles":bool
  in  "flag_serbia_montenegro":bool
  in  "flag_senegal":bool
  in  "flag_scotland":bool
  in  "flag_saudi_arabia":bool
  in  "flag_sao_tome_and_principe":bool
  in  "flag_san_marino":bool
  in  "flag_samoa":bool
  in  "flag_saint_vincent_and_grenadines":bool
  in  "flag_saint_pierre_and_miquelon":bool
  in  "flag_saint_lucia":bool
  in  "flag_saint_kitts_and_nevis":bool
  in  "flag_saint_helena":bool
  in  "flag_rwanda":bool
  in  "flag_russia":bool
  in  "flag_romania":bool
  in  "flag_red_cross":bool
  in  "flag_red":bool
  in  "flag_qatar":bool
  in  "flag_purple":bool
  in  "flag_puerto_rico":bool
  in  "flag_portugal":bool
  in  "flag_poland":bool
  in  "flag_pitcairn_islands":bool
  in  "flag_pink":bool
  in  "flag_philippines":bool
  in  "flag_peru":bool
  in  "flag_paraquay":bool
  in  "flag_papua_new_guinea":bool
  in  "flag_panama":bool
  in  "flag_palau":bool
  in  "flag_pakistan":bool
  in  "flag_orange":bool
  in  "flag_oman":bool
  in  "flag_olympic":bool
  in  "flag_norway":bool
  in  "flag_northern_mariana_islands":bool
  in  "flag_north_korea":bool
  in  "flag_norfolk_islands":bool
  in  "flag_niue":bool
  in  "flag_nigeria":bool
  in  "flag_niger":bool
  in  "flag_nicaragua":bool
  in  "flag_new_zealand":bool
  in  "flag_new":bool
  in  "flag_netherlands_antilles":bool
  in  "flag_netherlands":bool
  in  "flag_nepal":bool
  in  "flag_nauru":bool
  in  "flag_nato":bool
  in  "flag_namibia":bool
  in  "flag_mozambique":bool
  in  "flag_morocco":bool
  in  "flag_montserrat":bool
  in  "flag_mongolia":bool
  in  "flag_monaco":bool
  in  "flag_moldova":bool
  in  "flag_micronesia":bool
  in  "flag_mexico":bool
  in  "flag_mauritius":bool
  in  "flag_mauretania":bool
  in  "flag_martinique":bool
  in  "flag_marshall_islands":bool
  in  "flag_malta":bool
  in  "flag_mali":bool
  in  "flag_maledives":bool
  in  "flag_malaysia":bool
  in  "flag_malawi":bool
  in  "flag_madagascar":bool
  in  "flag_macedonia":bool
  in  "flag_macau":bool
  in  "flag_luxembourg":bool
  in  "flag_lithuania":bool
  in  "flag_liechtenstein":bool
  in  "flag_libya":bool
  in  "flag_liberia":bool
  in  "flag_lesotho":bool
  in  "flag_lebanon":bool
  in  "flag_latvia":bool
  in  "flag_laos":bool
  in  "flag_kyrgyzstan":bool
  in  "flag_kuwait":bool
  in  "flag_kiribati":bool
  in  "flag_kenya":bool
  in  "flag_kazakhstan":bool
  in  "flag_jordan":bool
  in  "flag_jersey":bool
  in  "flag_japan":bool
  in  "flag_jamaica":bool
  in  "flag_italy":bool
  in  "flag_israel":bool
  in  "flag_isle_of_man":bool
  in  "flag_ireland":bool
  in  "flag_iraq":bool
  in  "flag_iran":bool
  in  "flag_indonesia":bool
  in  "flag_india":bool
  in  "flag_iceland":bool
  in  "flag_hungary":bool
  in  "flag_hot":bool
  in  "flag_hong_kong":bool
  in  "flag_honduras":bool
  in  "flag_haiti":bool
  in  "flag_guyana":bool
  in  "flag_guinea_bissau":bool
  in  "flag_guinea":bool
  in  "flag_guernsey":bool
  in  "flag_guatemala":bool
  in  "flag_guam":bool
  in  "flag_grenada":bool
  in  "flag_greenland":bool
  in  "flag_green":bool
  in  "flag_greece":bool
  in  "flag_great_britain":bool
  in  "flag_gibraltar":bool
  in  "flag_ghana":bool
  in  "flag_germany":bool
  in  "flag_georgia":bool
  in  "flag_gambia":bool
  in  "flag_gabon":bool
  in  "flag_french_polynesia":bool
  in  "flag_france":bool
  in  "flag_finland":bool
  in  "flag_finish":bool
  in  "flag_fiji":bool
  in  "flag_faroe_islands":bool
  in  "flag_falkland_islands":bool
  in  "flag_european_union":bool
  in  "flag_ethiopia":bool
  in  "flag_estonia":bool
  in  "flag_eritrea":bool
  in  "flag_equatorial_guinea":bool
  in  "flag_equador":bool
  in  "flag_england":bool
  in  "flag_el_salvador":bool
  in  "flag_egypt":bool
  in  "flag_east_timor":bool
  in  "flag_dominican_republic":bool
  in  "flag_dominica":bool
  in  "flag_djibouti":bool
  in  "flag_denmark":bool
  in  "flag_czech_republic":bool
  in  "flag_cyprus":bool
  in  "flag_cuba":bool
  in  "flag_croatia":bool
  in  "flag_cote_divoire":bool
  in  "flag_costa_rica":bool
  in  "flag_cope_verde":bool
  in  "flag_cook_islands":bool
  in  "flag_congo_republic":bool
  in  "flag_congo_democratic_republic":bool
  in  "flag_comoros":bool
  in  "flag_colombia":bool
  in  "flag_china":bool
  in  "flag_chile":bool
  in  "flag_chad":bool
  in  "flag_central_african_republic":bool
  in  "flag_cayman_islands":bool
  in  "flag_canada":bool
  in  "flag_cameroon":bool
  in  "flag_cambodia":bool
  in  "flag_burundi":bool
  in  "flag_burma":bool
  in  "flag_burkina_faso":bool
  in  "flag_bulgaria":bool
  in  "flag_brunei":bool
  in  "flag_british_virgin_islands":bool
  in  "flag_british_indian_ocean":bool
  in  "flag_brazil":bool
  in  "flag_boy_scout":bool
  in  "flag_botswana":bool
  in  "flag_bosnia":bool
  in  "flag_bolivia":bool
  in  "flag_blue":bool
  in  "flag_bhutan":bool
  in  "flag_bermuda":bool
  in  "flag_benin":bool
  in  "flag_belize":bool
  in  "flag_belgium":bool
  in  "flag_belarus":bool
  in  "flag_barbados":bool
  in  "flag_bangladesh":bool
  in  "flag_bahrain":bool
  in  "flag_bahamas":bool
  in  "flag_azerbaijan":bool
  in  "flag_austria":bool
  in  "flag_australia":bool
  in  "flag_aruba":bool
  in  "flag_armenia":bool
  in  "flag_argentina":bool
  in  "flag_antigua_and_barbuda":bool
  in  "flag_anguilla":bool
  in  "flag_angola":bool
  in  "flag_andorra":bool
  in  "flag_american_samoa":bool
  in  "flag_algeria":bool
  in  "flag_albania":bool
  in  "flag_airfield_vehicle_safety":bool
  in  "flag_afghanistan":bool
  in  "flag_3":bool
  in  "flag_2":bool
  in  "flag_1":bool
  in  "fishfinder":bool
  in  "firewall_burn":bool
  in  "firewall":bool
  in  "firefox":bool
  in  "fire_extinguisher":bool
  in  "fire_damage":bool
  in  "fire":bool
  in  "fingerprint":bool
  in  "find":bool
  in  "finance":bool
  in  "filter_delete":bool
  in  "filter_add":bool
  in  "filter":bool
  in  "film_save":bool
  in  "film_photo":bool
  in  "film_link":bool
  in  "film_key":bool
  in  "film_go":bool
  in  "film_error":bool
  in  "film_edit":bool
  in  "film_delete":bool
  in  "film_add":bool
  in  "film":bool
  in  "fill":bool
  in  "file_manager":bool
  in  "file_extension_zip":bool
  in  "file_extension_xpi":bool
  in  "file_extension_xls":bool
  in  "file_extension_wps":bool
  in  "file_extension_wmv":bool
  in  "file_extension_wma":bool
  in  "file_extension_wav":bool
  in  "file_extension_vob":bool
  in  "file_extension_vcd":bool
  in  "file_extension_txt":bool
  in  "file_extension_ttf":bool
  in  "file_extension_torrent":bool
  in  "file_extension_tmp":bool
  in  "file_extension_tif":bool
  in  "file_extension_thm":bool
  in  "file_extension_tgz":bool
  in  "file_extension_swf":bool
  in  "file_extension_ss":bool
  in  "file_extension_sitx":bool
  in  "file_extension_sit":bool
  in  "file_extension_ses":bool
  in  "file_extension_sea":bool
  in  "file_extension_rtf":bool
  in  "file_extension_rmvb":bool
  in  "file_extension_rm":bool
  in  "file_extension_rar":bool
  in  "file_extension_ram":bool
  in  "file_extension_qxd":bool
  in  "file_extension_qbw":bool
  in  "file_extension_qbb":bool
  in  "file_extension_pub":bool
  in  "file_extension_ptb":bool
  in  "file_extension_pst":bool
  in  "file_extension_psd":bool
  in  "file_extension_ps":bool
  in  "file_extension_pps":bool
  in  "file_extension_png":bool
  in  "file_extension_pdf":bool
  in  "file_extension_ogg":bool
  in  "file_extension_mswmm":bool
  in  "file_extension_msi":bool
  in  "file_extension_mpg":bool
  in  "file_extension_mpeg":bool
  in  "file_extension_mp4":bool
  in  "file_extension_mp2":bool
  in  "file_extension_mov":bool
  in  "file_extension_mid":bool
  in  "file_extension_mdb":bool
  in  "file_extension_mcd":bool
  in  "file_extension_m4v":bool
  in  "file_extension_m4p":bool
  in  "file_extension_m4b":bool
  in  "file_extension_m4a":bool
  in  "file_extension_log":bool
  in  "file_extension_lnk":bool
  in  "file_extension_jpg":bool
  in  "file_extension_jpeg":bool
  in  "file_extension_jar":bool
  in  "file_extension_iso":bool
  in  "file_extension_indd":bool
  in  "file_extension_ifo":bool
  in  "file_extension_html":bool
  in  "file_extension_htm":bool
  in  "file_extension_hqx":bool
  in  "file_extension_gz":bool
  in  "file_extension_gif":bool
  in  "file_extension_flv":bool
  in  "file_extension_fla":bool
  in  "file_extension_exe":bool
  in  "file_extension_eps":bool
  in  "file_extension_eml":bool
  in  "file_extension_dwg":bool
  in  "file_extension_dvf":bool
  in  "file_extension_dss":bool
  in  "file_extension_doc":bool
  in  "file_extension_dmg":bool
  in  "file_extension_dll":bool
  in  "file_extension_divx":bool
  in  "file_extension_dat":bool
  in  "file_extension_chm":bool
  in  "file_extension_cdr":bool
  in  "file_extension_cdl":bool
  in  "file_extension_cda":bool
  in  "file_extension_cbr":bool
  in  "file_extension_cab":bool
  in  "file_extension_bup":bool
  in  "file_extension_bmp":bool
  in  "file_extension_bin":bool
  in  "file_extension_bat":bool
  in  "file_extension_asx":bool
  in  "file_extension_asf":bool
  in  "file_extension_amr":bool
  in  "file_extension_aiff":bool
  in  "file_extension_aif":bool
  in  "file_extension_ai":bool
  in  "file_extension_ace":bool
  in  "file_extension_7z":bool
  in  "file_extension_3gp":bool
  in  "female":bool
  in  "feed_magnify":bool
  in  "feed_key":bool
  in  "feed_go":bool
  in  "feed_error":bool
  in  "feed_edit":bool
  in  "feed_disk":bool
  in  "feed_delete":bool
  in  "feed_add":bool
  in  "feed":bool
  in  "fedora":bool
  in  "fax":bool
  in  "fatcow":bool
  in  "factory":bool
  in  "facebook":bool
  in  "faberge_egg":bool
  in  "eye_red":bool
  in  "eye_close":bool
  in  "eye":bool
  in  "extract_foreground_objects":bool
  in  "external":bool
  in  "export_excel":bool
  in  "exclamation":bool
  in  "evernote":bool
  in  "events":bool
  in  "evacuator":bool
  in  "escimo_pie":bool
  in  "error_go":bool
  in  "error_delete":bool
  in  "error_add":bool
  in  "error":bool
  in  "envelope_string":bool
  in  "envelope":bool
  in  "entity":bool
  in  "emotion_zedz":bool
  in  "emotion_wink":bool
  in  "emotion_whist":bool
  in  "emotion_what":bool
  in  "emotion_waii":bool
  in  "emotion_waaaht":bool
  in  "emotion_vampire":bool
  in  "emotion_unshaven":bool
  in  "emotion_unhappy":bool
  in  "emotion_too_sad":bool
  in  "emotion_tongue":bool
  in  "emotion_tire":bool
  in  "emotion_terminator":bool
  in  "emotion_sweat":bool
  in  "emotion_surrender":bool
  in  "emotion_sure":bool
  in  "emotion_suprised":bool
  in  "emotion_stupid":bool
  in  "emotion_star":bool
  in  "emotion_spy":bool
  in  "emotion_spiderman":bool
  in  "emotion_smile":bool
  in  "emotion_sleep":bool
  in  "emotion_skull":bool
  in  "emotion_silent":bool
  in  "emotion_sick":bool
  in  "emotion_shocked":bool
  in  "emotion_shame":bool
  in  "emotion_sad":bool
  in  "emotion_red":bool
  in  "emotion_rap":bool
  in  "emotion_question":bool
  in  "emotion_pumpkin":bool
  in  "emotion_pirate":bool
  in  "emotion_nosebleed":bool
  in  "emotion_ninja":bool
  in  "emotion_nerd":bool
  in  "emotion_mummy":bool
  in  "emotion_money":bool
  in  "emotion_misdoubt":bool
  in  "emotion_medic":bool
  in  "emotion_matrix":bool
  in  "emotion_mad":bool
  in  "emotion_love":bool
  in  "emotion_kissed":bool
  in  "emotion_kiss":bool
  in  "emotion_jason":bool
  in  "emotion_japan":bool
  in  "emotion_hypnotized":bool
  in  "emotion_hungry":bool
  in  "emotion_horror":bool
  in  "emotion_hitler":bool
  in  "emotion_happy":bool
  in  "emotion_hand_flower":bool
  in  "emotion_haha":bool
  in  "emotion_grin":bool
  in  "emotion_greedy":bool
  in  "emotion_go":bool
  in  "emotion_girl":bool
  in  "emotion_ghost":bool
  in  "emotion_gear":bool
  in  "emotion_franken":bool
  in  "emotion_flower_dead":bool
  in  "emotion_fan":bool
  in  "emotion_face_panda":bool
  in  "emotion_face_monkey":bool
  in  "emotion_eyes_droped":bool
  in  "emotion_exciting":bool
  in  "emotion_evolution":bool
  in  "emotion_evilgrin":bool
  in  "emotion_dribble":bool
  in  "emotion_doubt":bool
  in  "emotion_diver":bool
  in  "emotion_devil":bool
  in  "emotion_dead":bool
  in  "emotion_david_blaine":bool
  in  "emotion_darth_wader":bool
  in  "emotion_cyclops":bool
  in  "emotion_cry":bool
  in  "emotion_crazy_rabbit":bool
  in  "emotion_crazy":bool
  in  "emotion_cool":bool
  in  "emotion_confuse":bool
  in  "emotion_confident":bool
  in  "emotion_cold":bool
  in  "emotion_clown":bool
  in  "emotion_bye_bye":bool
  in  "emotion_bubblegum":bool
  in  "emotion_bloody":bool
  in  "emotion_bigsmile":bool
  in  "emotion_beaten":bool
  in  "emotion_beat_brick":bool
  in  "emotion_batman":bool
  in  "emotion_baffle":bool
  in  "emotion_bad_smelly":bool
  in  "emotion_bad_egg":bool
  in  "emotion_baby":bool
  in  "emotion_angry":bool
  in  "emotion_anger":bool
  in  "emotion_angel":bool
  in  "emotion_amazing":bool
  in  "emotion_alien":bool
  in  "emotion_ah":bool
  in  "emotion_after_boom":bool
  in  "emotion_adore":bool
  in  "ember":bool
  in  "emails_stack":bool
  in  "emails":bool
  in  "email_to_friend":bool
  in  "email_send_receive":bool
  in  "email_open_image":bool
  in  "email_open":bool
  in  "email_link":bool
  in  "email_go":bool
  in  "email_forward":bool
  in  "email_error":bool
  in  "email_edit":bool
  in  "email_delete":bool
  in  "email_attach":bool
  in  "email_at_sign":bool
  in  "email_air":bool
  in  "email_add":bool
  in  "email":bool
  in  "elements":bool
  in  "electric_guitar":bool
  in  "ehow":bool
  in  "egyptian_pyramid":bool
  in  "education":bool
  in  "edit_path":bool
  in  "edit_mathematics":bool
  in  "edit_free":bool
  in  "edit_diff":bool
  in  "edit_chain":bool
  in  "echeck":bool
  in  "ebay":bool
  in  "earth_night":bool
  in  "ear_listen":bool
  in  "e_book_reader_white":bool
  in  "e_book_reader_black":bool
  in  "dynamite":bool
  in  "dvd_link":bool
  in  "dvd_key":bool
  in  "dvd_go":bool
  in  "dvd_error":bool
  in  "dvd_edit":bool
  in  "dvd_delete":bool
  in  "dvd_add":bool
  in  "dvd":bool
  in  "drum":bool
  in  "drugs_com":bool
  in  "drop":bool
  in  "drive_web":bool
  in  "drive_user":bool
  in  "drive_rename":bool
  in  "drive_network":bool
  in  "drive_magnify":bool
  in  "drive_link":bool
  in  "drive_key":bool
  in  "drive_go":bool
  in  "drive_error":bool
  in  "drive_edit":bool
  in  "drive_disk":bool
  in  "drive_delete":bool
  in  "drive_cd_empty":bool
  in  "drive_cd":bool
  in  "drive_burn":bool
  in  "drive_add":bool
  in  "drive":bool
  in  "drink_empty":bool
  in  "drink":bool
  in  "drill":bool
  in  "dribbble":bool
  in  "drawer_open":bool
  in  "drawer":bool
  in  "draw_wave":bool
  in  "draw_vertex":bool
  in  "draw_star":bool
  in  "draw_spiral":bool
  in  "draw_smudge":bool
  in  "draw_ring":bool
  in  "draw_polyline":bool
  in  "draw_polygon_curves":bool
  in  "draw_polygon":bool
  in  "draw_points":bool
  in  "draw_path":bool
  in  "draw_line":bool
  in  "draw_island":bool
  in  "draw_ink":bool
  in  "draw_eraser":bool
  in  "draw_ellipse":bool
  in  "draw_dodge_burn":bool
  in  "draw_convolve":bool
  in  "draw_clone":bool
  in  "draw_calligraphic":bool
  in  "draw_airbrush":bool
  in  "download_for_windows":bool
  in  "download_for_mac":bool
  in  "download_for_linux":bool
  in  "download_cloud":bool
  in  "download":bool
  in  "down_jacket":bool
  in  "dopplr":bool
  in  "door_out":bool
  in  "door_open":bool
  in  "door_in":bool
  in  "door":bool
  in  "donut":bool
  in  "domain_template":bool
  in  "domain_names_advanced":bool
  in  "domain_name_monetization":bool
  in  "domain_name_investment":bool
  in  "domain_legal_issues":bool
  in  "domain_controversies":bool
  in  "domain_buying_selling":bool
  in  "dog":bool
  in  "documents_email":bool
  in  "document_yellow":bool
  in  "document_white_torn":bool
  in  "document_view_book":bool
  in  "document_vertical":bool
  in  "document_valid":bool
  in  "document_tree":bool
  in  "document_torn":bool
  in  "document_todo":bool
  in  "document_tag":bool
  in  "document_stand":bool
  in  "document_split":bool
  in  "document_spacing":bool
  in  "document_signature":bool
  in  "document_shred":bool
  in  "document_shapes":bool
  in  "document_rename":bool
  in  "document_redirect":bool
  in  "document_red":bool
  in  "document_quote":bool
  in  "document_properties":bool
  in  "document_prepare":bool
  in  "document_plus":bool
  in  "document_page_previous":bool
  in  "document_page_next":bool
  in  "document_page_last":bool
  in  "document_page":bool
  in  "document_num":bool
  in  "document_notes":bool
  in  "document_next":bool
  in  "document_move":bool
  in  "document_mark_as_final":bool
  in  "document_margins":bool
  in  "document_layout":bool
  in  "document_inspector":bool
  in  "document_inspect":bool
  in  "document_insert":bool
  in  "document_info":bool
  in  "document_index":bool
  in  "document_import":bool
  in  "document_image_ver":bool
  in  "document_image_hor":bool
  in  "document_image":bool
  in  "document_green":bool
  in  "document_font_wizard":bool
  in  "document_font":bool
  in  "document_export":bool
  in  "document_empty":bool
  in  "document_editing":bool
  in  "document_copies":bool
  in  "document_comments":bool
  in  "document_comment_below":bool
  in  "document_comment_behind":bool
  in  "document_comment_above":bool
  in  "document_check_compatibility":bool
  in  "document_center":bool
  in  "document_break":bool
  in  "document_black":bool
  in  "document_background":bool
  in  "document_back":bool
  in  "do_not_disturb":bool
  in  "dns_setting":bool
  in  "dns":bool
  in  "distribution_partnerships":bool
  in  "disk_multiple":bool
  in  "disk":bool
  in  "dish":bool
  in  "discover":bool
  in  "disconnect":bool
  in  "directory_listing":bool
  in  "direction":bool
  in  "dinersclub":bool
  in  "digital_signature_pen":bool
  in  "digital_signature":bool
  in  "digg":bool
  in  "dice":bool
  in  "diamond":bool
  in  "dialog":bool
  in  "diagramm":bool
  in  "diagnostic_chart":bool
  in  "devianart":bool
  in  "desktop":bool
  in  "designmoo":bool
  in  "design_float":bool
  in  "derivatives":bool
  in  "delicious":bool
  in  "delete":bool
  in  "decimal_more":bool
  in  "decimal_less":bool
  in  "debian":bool
  in  "ddr_memory":bool
  in  "date_task":bool
  in  "date_relation":bool
  in  "date_previous_gray":bool
  in  "date_previous":bool
  in  "date_next_gray":bool
  in  "date_next":bool
  in  "date_magnify":bool
  in  "date_link":bool
  in  "date_go":bool
  in  "date_error":bool
  in  "date_edit":bool
  in  "date_delete":bool
  in  "date_add":bool
  in  "date":bool
  in  "database_yellow":bool
  in  "database_table":bool
  in  "database_server":bool
  in  "database_save":bool
  in  "database_refresh":bool
  in  "database_red":bool
  in  "database_link":bool
  in  "database_lightning":bool
  in  "database_key":bool
  in  "database_green":bool
  in  "database_go":bool
  in  "database_gear":bool
  in  "database_error":bool
  in  "database_edit":bool
  in  "database_delete":bool
  in  "database_connect":bool
  in  "database_blue":bool
  in  "database_black":bool
  in  "database_add":bool
  in  "database":bool
  in  "data_table":bool
  in  "data_sort":bool
  in  "data_grid":bool
  in  "data_field":bool
  in  "data_chooser":bool
  in  "dashboard":bool
  in  "cutter":bool
  in  "cutlery":bool
  in  "cutleries":bool
  in  "cut_red":bool
  in  "cut":bool
  in  "cushion":bool
  in  "curtain":bool
  in  "cursor":bool
  in  "curriculum_vitae":bool
  in  "cup_silver":bool
  in  "cup_link":bool
  in  "cup_key":bool
  in  "cup_gold":bool
  in  "cup_go":bool
  in  "cup_error":bool
  in  "cup_edit":bool
  in  "cup_delete":bool
  in  "cup_bronze":bool
  in  "cup_add":bool
  in  "cup":bool
  in  "css_valid":bool
  in  "css_go":bool
  in  "css_delete":bool
  in  "css_add":bool
  in  "css_3":bool
  in  "css":bool
  in  "cruise_ship":bool
  in  "crown_silver":bool
  in  "crown_gold":bool
  in  "crown_bronze":bool
  in  "cross_shield":bool
  in  "cross_promotion_selling":bool
  in  "cross":bool
  in  "cricket":bool
  in  "creditcards":bool
  in  "credit":bool
  in  "creative_commons":bool
  in  "counter":bool
  in  "copyleft":bool
  in  "copying_and_distribution":bool
  in  "cooler":bool
  in  "cookies":bool
  in  "cookie_chocolate":bool
  in  "convert_gray_to_color":bool
  in  "convert_color_to_gray":bool
  in  "conversion_of_currency":bool
  in  "controller_error":bool
  in  "controller_delete":bool
  in  "controller_add":bool
  in  "controller":bool
  in  "controlbar":bool
  in  "control_stop_blue":bool
  in  "control_stop":bool
  in  "control_start_blue":bool
  in  "control_start":bool
  in  "control_rewind_blue":bool
  in  "control_rewind":bool
  in  "control_repeat_blue":bool
  in  "control_repeat":bool
  in  "control_power_blue":bool
  in  "control_power":bool
  in  "control_play_blue":bool
  in  "control_play":bool
  in  "control_pause_record":bool
  in  "control_pause_blue":bool
  in  "control_pause":bool
  in  "control_panel_branding":bool
  in  "control_panel_access":bool
  in  "control_panel":bool
  in  "control_fastforward_blue":bool
  in  "control_fastforward":bool
  in  "control_equalizer_blue":bool
  in  "control_equalizer":bool
  in  "control_end_blue":bool
  in  "control_end":bool
  in  "control_eject_blue":bool
  in  "control_eject":bool
  in  "control_cursor_blue":bool
  in  "control_cursor":bool
  in  "contrast_low":bool
  in  "contrast_increase":bool
  in  "contrast_high":bool
  in  "contrast_decrease":bool
  in  "contrast":bool
  in  "contact_email":bool
  in  "construction":bool
  in  "connect":bool
  in  "computer_link":bool
  in  "computer_key":bool
  in  "computer_go":bool
  in  "computer_error":bool
  in  "computer_edit":bool
  in  "computer_delete":bool
  in  "computer_add":bool
  in  "computer":bool
  in  "compress":bool
  in  "compile_warning":bool
  in  "compile_error":bool
  in  "compile":bool
  in  "compass":bool
  in  "company_generosity":bool
  in  "comments_twitter":bool
  in  "comments_facebook":bool
  in  "comments_delete":bool
  in  "comments_add":bool
  in  "comments":bool
  in  "comment_white":bool
  in  "comment_twitter_retwit":bool
  in  "comment_twitter_box":bool
  in  "comment_twitter":bool
  in  "comment_google":bool
  in  "comment_facebook_box":bool
  in  "comment_facebook":bool
  in  "comment_edit":bool
  in  "comment_delete":bool
  in  "comment_box":bool
  in  "comment_add":bool
  in  "comment":bool
  in  "combo_box":bool
  in  "columnchart":bool
  in  "column_two":bool
  in  "column_tree":bool
  in  "column_single":bool
  in  "column_right":bool
  in  "column_one":bool
  in  "column_left":bool
  in  "column_four":bool
  in  "column_double":bool
  in  "color_wheel":bool
  in  "color_swatches":bool
  in  "color_swatch":bool
  in  "color_picker_alternative":bool
  in  "color_picker":bool
  in  "color_management":bool
  in  "color_gradient":bool
  in  "color_adjustment_red":bool
  in  "color_adjustment_green":bool
  in  "color_adjustment_blue":bool
  in  "color_adjustment":bool
  in  "cold":bool
  in  "coins_in_hand":bool
  in  "coins_delete":bool
  in  "coins_add":bool
  in  "coins":bool
  in  "coin_stack_gold":bool
  in  "coin_single_silver":bool
  in  "coin_single_gold":bool
  in  "coin_single_cooper":bool
  in  "cog_go":bool
  in  "cog_error":bool
  in  "cog_edit":bool
  in  "cog_delete":bool
  in  "cog_add":bool
  in  "cog":bool
  in  "code":bool
  in  "cocacola":bool
  in  "co2":bool
  in  "clown_fish":bool
  in  "clock_stop":bool
  in  "clock_select_remain":bool
  in  "clock_red":bool
  in  "clock_play":bool
  in  "clock_pause":bool
  in  "clock_moon_phase":bool
  in  "clock_link":bool
  in  "clock_history_frame":bool
  in  "clock_go":bool
  in  "clock_error":bool
  in  "clock_edit":bool
  in  "clock_delete":bool
  in  "clock_add":bool
  in  "clock_45":bool
  in  "clock_15":bool
  in  "clock":bool
  in  "clipboard_sign_out":bool
  in  "clipboard_sign":bool
  in  "clipboard_invoice":bool
  in  "clipboard_empty":bool
  in  "clip_splitter":bool
  in  "client_account_template":bool
  in  "cirrus":bool
  in  "circus":bool
  in  "cinema_ticket":bool
  in  "cigarette":bool
  in  "church":bool
  in  "christmas_tree":bool
  in  "chocolate_bite":bool
  in  "chocolate":bool
  in  "chinese_noodles":bool
  in  "children_cap":bool
  in  "chiken_leg":bool
  in  "chess_tower":bool
  in  "chess_horse":bool
  in  "cheque":bool
  in  "chefs_hat":bool
  in  "cheese":bool
  in  "checkerboard":bool
  in  "check_box":bool
  in  "chartplotter":bool
  in  "chart_up_color":bool
  in  "chart_stock":bool
  in  "chart_pie_link":bool
  in  "chart_pie_error":bool
  in  "chart_pie_edit":bool
  in  "chart_pie_delete":bool
  in  "chart_pie_alternative":bool
  in  "chart_pie_add":bool
  in  "chart_pie":bool
  in  "chart_organisation_delete":bool
  in  "chart_organisation_add":bool
  in  "chart_organisation":bool
  in  "chart_line_link":bool
  in  "chart_line_error":bool
  in  "chart_line_edit":bool
  in  "chart_line_delete":bool
  in  "chart_line_add":bool
  in  "chart_line":bool
  in  "chart_down_color":bool
  in  "chart_curve_link":bool
  in  "chart_curve_go":bool
  in  "chart_curve_error":bool
  in  "chart_curve_edit":bool
  in  "chart_curve_delete":bool
  in  "chart_curve_add":bool
  in  "chart_curve":bool
  in  "chart_column_2":bool
  in  "chart_column":bool
  in  "chart_bullseye":bool
  in  "chart_bar_link":bool
  in  "chart_bar_error":bool
  in  "chart_bar_edit":bool
  in  "chart_bar_delete":bool
  in  "chart_bar_add":bool
  in  "chart_bar":bool
  in  "change_password":bool
  in  "chameleon":bool
  in  "chair":bool
  in  "ceo":bool
  in  "centroid":bool
  in  "centos":bool
  in  "celsius":bool
  in  "cd_go":bool
  in  "cd_eject":bool
  in  "cd_edit":bool
  in  "cd_delete":bool
  in  "cd_case_empty":bool
  in  "cd_case":bool
  in  "cd_burn":bool
  in  "cd_add":bool
  in  "cd":bool
  in  "cctv_camera":bool
  in  "caution_radiation":bool
  in  "caution_high_voltage":bool
  in  "caution_board":bool
  in  "caution_biohazard":bool
  in  "cats_display":bool
  in  "caterpillar":bool
  in  "category_item_select":bool
  in  "category_item":bool
  in  "category_group_select":bool
  in  "category_group":bool
  in  "category":bool
  in  "categories":bool
  in  "cat":bool
  in  "cash_terminal":bool
  in  "cash_stack":bool
  in  "cash_register_2":bool
  in  "cash_register":bool
  in  "cart_remove":bool
  in  "cart_put":bool
  in  "cart_go":bool
  in  "cart_full":bool
  in  "cart_error":bool
  in  "cart_edit":bool
  in  "cart_delete":bool
  in  "cart_add":bool
  in  "cart":bool
  in  "cargo":bool
  in  "cards_binds":bool
  in  "cards_bind_address":bool
  in  "cards":bool
  in  "card_solo":bool
  in  "card_save":bool
  in  "card_sapphire":bool
  in  "card_money":bool
  in  "card_miles":bool
  in  "card_ipod":bool
  in  "card_import":bool
  in  "card_gold":bool
  in  "card_gift_2":bool
  in  "card_gift":bool
  in  "card_front":bool
  in  "card_export":bool
  in  "card_echeck":bool
  in  "card_discover_novus":bool
  in  "card_discover_black":bool
  in  "card_debit":bool
  in  "card_credit":bool
  in  "card_chip_silver":bool
  in  "card_chip_gold":bool
  in  "card_chase":bool
  in  "card_bank":bool
  in  "card_back":bool
  in  "card_apple":bool
  in  "card_amex_green":bool
  in  "card_amex_gray":bool
  in  "card_amex_gold":bool
  in  "card_amazon":bool
  in  "car_taxi":bool
  in  "car_delete":bool
  in  "car_add":bool
  in  "car":bool
  in  "cap":bool
  in  "canvas_size":bool
  in  "canvas":bool
  in  "candy_cane":bool
  in  "candlestickchart":bool
  in  "candle_2":bool
  in  "candle":bool
  in  "cancel":bool
  in  "camera_small":bool
  in  "camera_link":bool
  in  "camera_lens":bool
  in  "camera_go":bool
  in  "camera_error":bool
  in  "camera_edit":bool
  in  "camera_delete":bool
  in  "camera_black":bool
  in  "camera_add":bool
  in  "camera":bool
  in  "camcorder":bool
  in  "calendar_view_week":bool
  in  "calendar_view_month":bool
  in  "calendar_view_day":bool
  in  "calendar_link":bool
  in  "calendar_edit":bool
  in  "calendar_delete":bool
  in  "calendar_copy":bool
  in  "calendar_add":bool
  in  "calendar":bool
  in  "calculator_link":bool
  in  "calculator_error":bool
  in  "calculator_edit":bool
  in  "calculator_delete":bool
  in  "calculator_black":bool
  in  "calculator_add":bool
  in  "calculator":bool
  in  "cake":bool
  in  "cactus":bool
  in  "buzz":bool
  in  "buttonbar":bool
  in  "button":bool
  in  "butterfly":bool
  in  "bus":bool
  in  "burro":bool
  in  "bullet_yellow":bool
  in  "bullet_wrench":bool
  in  "bullet_world":bool
  in  "bullet_word":bool
  in  "bullet_white":bool
  in  "bullet_vector":bool
  in  "bullet_valid":bool
  in  "bullet_user":bool
  in  "bullet_up":bool
  in  "bullet_toggle_plus":bool
  in  "bullet_toggle_minus":bool
  in  "bullet_textfield":bool
  in  "bullet_table":bool
  in  "bullet_star":bool
  in  "bullet_red":bool
  in  "bullet_purple":bool
  in  "bullet_powerpoint":bool
  in  "bullet_pink":bool
  in  "bullet_picture":bool
  in  "bullet_php":bool
  in  "bullet_palette":bool
  in  "bullet_orange":bool
  in  "bullet_office":bool
  in  "bullet_medal":bool
  in  "bullet_magnify":bool
  in  "bullet_link":bool
  in  "bullet_lightning":bool
  in  "bullet_key":bool
  in  "bullet_green":bool
  in  "bullet_go":bool
  in  "bullet_gear":bool
  in  "bullet_flash":bool
  in  "bullet_find":bool
  in  "bullet_feed":bool
  in  "bullet_excel":bool
  in  "bullet_error":bool
  in  "bullet_edit":bool
  in  "bullet_dvd":bool
  in  "bullet_down":bool
  in  "bullet_document":bool
  in  "bullet_disk":bool
  in  "bullet_delete":bool
  in  "bullet_database":bool
  in  "bullet_connect":bool
  in  "bullet_code_red":bool
  in  "bullet_code":bool
  in  "bullet_chart":bool
  in  "bullet_cd":bool
  in  "bullet_camera":bool
  in  "bullet_burn":bool
  in  "bullet_bulb_on":bool
  in  "bullet_bulb_off":bool
  in  "bullet_bug":bool
  in  "bullet_brush":bool
  in  "bullet_blue":bool
  in  "bullet_black":bool
  in  "bullet_bell":bool
  in  "bullet_back":bool
  in  "bullet_attach":bool
  in  "bullet_arrow_up":bool
  in  "bullet_arrow_top":bool
  in  "bullet_arrow_right_2":bool
  in  "bullet_arrow_right":bool
  in  "bullet_arrow_left_2":bool
  in  "bullet_arrow_left":bool
  in  "bullet_arrow_down":bool
  in  "bullet_arrow_bottom":bool
  in  "bullet_archive":bool
  in  "bullet_add":bool
  in  "bulb":bool
  in  "building_link":bool
  in  "building_key":bool
  in  "building_go":bool
  in  "building_error":bool
  in  "building_edit":bool
  in  "building_delete":bool
  in  "building_add":bool
  in  "building":bool
  in  "bug_link":bool
  in  "bug_go":bool
  in  "bug_error":bool
  in  "bug_edit":bool
  in  "bug_delete":bool
  in  "bug_add":bool
  in  "bug":bool
  in  "bucket_truck":bool
  in  "bubblechart":bool
  in  "brushes":bool
  in  "broom":bool
  in  "brightkite":bool
  in  "briefcase":bool
  in  "bricks":bool
  in  "brick_link":bool
  in  "brick_go":bool
  in  "brick_error":bool
  in  "brick_edit":bool
  in  "brick_delete":bool
  in  "brick_add":bool
  in  "brick":bool
  in  "breeze":bool
  in  "bread":bool
  in  "brain_trainer":bool
  in  "brain":bool
  in  "boxing_glove":bool
  in  "box_search":bool
  in  "box_open":bool
  in  "box_front":bool
  in  "box_down":bool
  in  "box_closed":bool
  in  "box":bool
  in  "bow":bool
  in  "border_color":bool
  in  "border_2_top":bool
  in  "border_2_right":bool
  in  "border_2_outer":bool
  in  "border_2_left":bool
  in  "border_2_bottom":bool
  in  "border_1d_top":bool
  in  "border_1d_right":bool
  in  "border_1d_left":bool
  in  "border_1d_bottom":bool
  in  "border_1d_around":bool
  in  "border_1_ver":bool
  in  "border_1_top":bool
  in  "border_1_right":bool
  in  "border_1_outer":bool
  in  "border_1_none":bool
  in  "border_1_middle":bool
  in  "border_1_left":bool
  in  "border_1_hor":bool
  in  "border_1_bottom":bool
  in  "border_1":bool
  in  "boomerang":bool
  in  "bookshelf":bool
  in  "books_stack":bool
  in  "books":bool
  in  "bookmark_red":bool
  in  "bookmark":bool
  in  "book_spelling":bool
  in  "book_previous":bool
  in  "book_picture":bool
  in  "book_open":bool
  in  "book_next":bool
  in  "book_link":bool
  in  "book_key":bool
  in  "book_keeping":bool
  in  "book_go":bool
  in  "book_error":bool
  in  "book_edit":bool
  in  "book_delete":bool
  in  "book_addresses":bool
  in  "book_add":bool
  in  "book":bool
  in  "bomb":bool
  in  "board_game":bool
  in  "bluetooth":bool
  in  "blueprints":bool
  in  "blueprint_horizontal":bool
  in  "blueprint":bool
  in  "blogs":bool
  in  "blogger":bool
  in  "blackboard_sum":bool
  in  "blackboard_steps":bool
  in  "blackboard_empty":bool
  in  "blackboard_drawing":bool
  in  "blackberry_white":bool
  in  "blackberry_messenger":bool
  in  "blackberry":bool
  in  "bios":bool
  in  "bin_recycle":bool
  in  "bin_empty":bool
  in  "bin_closed":bool
  in  "bin":bool
  in  "billiard_marker":bool
  in  "bell_link":bool
  in  "bell_go":bool
  in  "bell_error":bool
  in  "bell_delete":bool
  in  "bell_add":bool
  in  "bell":bool
  in  "beer":bool
  in  "bedo":bool
  in  "bed":bool
  in  "bean":bool
  in  "beaker_empty":bool
  in  "beaker":bool
  in  "battery_plug":bool
  in  "battery_low":bool
  in  "battery_half":bool
  in  "battery_full":bool
  in  "battery_charge":bool
  in  "battery":bool
  in  "baton":bool
  in  "basket_remove":bool
  in  "basket_put":bool
  in  "basket_go":bool
  in  "basket_full":bool
  in  "basket_error":bool
  in  "basket_edit":bool
  in  "basket_delete":bool
  in  "basket_add":bool
  in  "basket":bool
  in  "barcode_2d":bool
  in  "barcode":bool
  in  "barchart":bool
  in  "bank":bool
  in  "bandaid":bool
  in  "bamboos":bool
  in  "bamboo":bool
  in  "baloon_2_empty":bool
  in  "baloon_2":bool
  in  "baloon":bool
  in  "ballon":bool
  in  "balance_unbalance":bool
  in  "balance":bool
  in  "baggage_cart_box":bool
  in  "baggage_cart":bool
  in  "backup_manager":bool
  in  "backpack":bool
  in  "baby_bottle":bool
  in  "ax":bool
  in  "award_star_silver_3":bool
  in  "award_star_silver_2":bool
  in  "award_star_silver_1":bool
  in  "award_star_gold_3":bool
  in  "award_star_gold_2":bool
  in  "award_star_gold_1":bool
  in  "award_star_delete":bool
  in  "award_star_bronze_3":bool
  in  "award_star_bronze_2":bool
  in  "award_star_bronze_1":bool
  in  "award_star_add":bool
  in  "autos":bool
  in  "auction_hammer_gavel":bool
  in  "attribution":bool
  in  "attributes_display":bool
  in  "attach":bool
  in  "atm":bool
  in  "at_sign":bool
  in  "asterisk_yellow":bool
  in  "asterisk_orange":bool
  in  "ask_and_answer":bool
  in  "artwork":bool
  in  "arrow_up":bool
  in  "arrow_undo":bool
  in  "arrow_turn_right":bool
  in  "arrow_turn_left":bool
  in  "arrow_switch":bool
  in  "arrow_rotate_clockwise":bool
  in  "arrow_rotate_anticlockwise":bool
  in  "arrow_right":bool
  in  "arrow_refresh_small":bool
  in  "arrow_refresh":bool
  in  "arrow_redo":bool
  in  "arrow_out":bool
  in  "arrow_merge":bool
  in  "arrow_left":bool
  in  "arrow_join":bool
  in  "arrow_inout":bool
  in  "arrow_in":bool
  in  "arrow_down":bool
  in  "arrow_divide":bool
  in  "arrow_branch":bool
  in  "areachart":bool
  in  "arch_linux":bool
  in  "application_xp_terminal":bool
  in  "application_xp":bool
  in  "application_view_tile":bool
  in  "application_view_list":bool
  in  "application_view_icons":bool
  in  "application_view_gallery":bool
  in  "application_view_detail":bool
  in  "application_view_columns":bool
  in  "application_tile_vertical":bool
  in  "application_tile_horizontal":bool
  in  "application_split":bool
  in  "application_side_tree":bool
  in  "application_side_list":bool
  in  "application_side_expand":bool
  in  "application_side_contract":bool
  in  "application_side_boxes":bool
  in  "application_put":bool
  in  "application_osx_terminal":bool
  in  "application_osx":bool
  in  "application_link":bool
  in  "application_lightning":bool
  in  "application_key":bool
  in  "application_home":bool
  in  "application_go":bool
  in  "application_get":bool
  in  "application_from_storage":bool
  in  "application_form_magnify":bool
  in  "application_form_edit":bool
  in  "application_form_delete":bool
  in  "application_form_add":bool
  in  "application_form":bool
  in  "application_error":bool
  in  "application_edit":bool
  in  "application_double":bool
  in  "application_delete":bool
  in  "application_control_bar":bool
  in  "application_cascade":bool
  in  "application_add":bool
  in  "application":bool
  in  "apple_half":bool
  in  "apple_corp":bool
  in  "apple":bool
  in  "aol_messenger":bool
  in  "aol_mail":bool
  in  "anti_xss":bool
  in  "angel":bool
  in  "android":bool
  in  "anchor":bool
  in  "american_express":bool
  in  "all_right_reserved":bool
  in  "alitalk":bool
  in  "align_right":bool
  in  "align_none":bool
  in  "align_middle":bool
  in  "align_left":bool
  in  "align_compact":bool
  in  "align_center":bool
  in  "align_bellow":bool
  in  "align_above":bool
  in  "alarm_bell":bool
  in  "aim_messenger":bool
  in  "agp":bool
  in  "advertising":bool
  in  "advanced_data_grid":bool
  in  "administrator":bool
  in  "add":bool
  in  "active_sessions":bool
  in  "action_log":bool
  in  "acoustic_guitar":bool
  in  "acorn":bool
  in  "account_balances":bool
  in  "accordion":bool
  in  "accept":bool
  in  "64_bit":bool
  in  "32_bit":bool
  in  "3d_glasses":bool
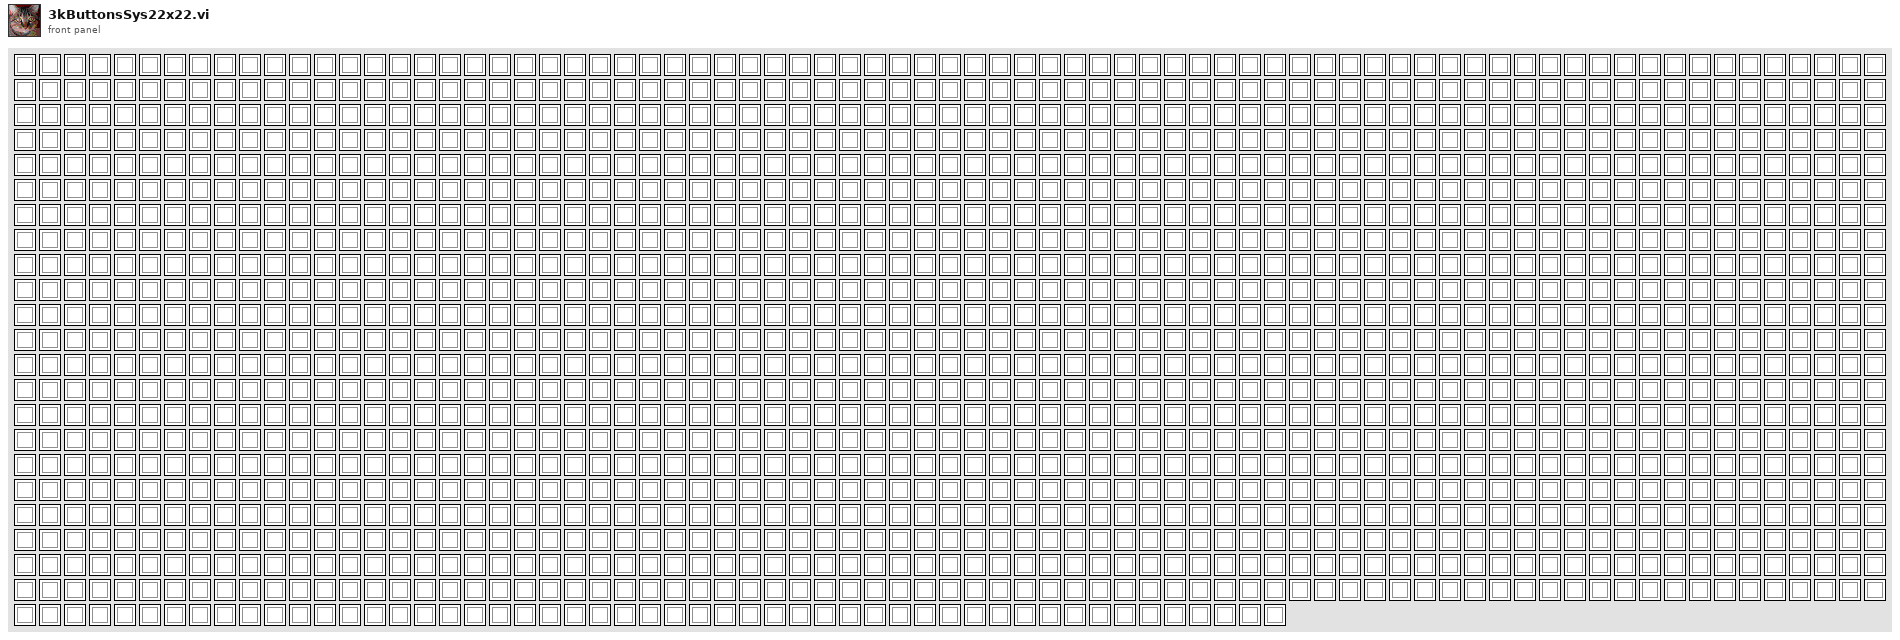
[diagram p1: front panel]
diagram:
